vi "tdms file.vi"   [LabVIEW 2020]
uses:
  Nominal Client/Nominal Client.lvclass/Nominal Client.ctl
  nominal types/workspace/workspace.lvclass/workspace.ctl
  7420467e-f5dd-4a0f-ae77-be3a0843df19.vi
  Nominal Client/private_data.set.vi
  7420467e-f5dd-4a0f-ae77-be3a0843df19.vi/8284acbc-2d4d-4b18-b492-8ff51a6e7e10.vi
  nominal types/workspace/id.get.vi
  nominal types/workspace/rid.get.vi
  <vilib>/AdvancedString/1D String Array to Delimited String.vi
  Nominal Client/workspace.set.vi
  <vilib>/Utility/error.llb/Error Cluster From Error Code.vi
  Nominal Client/format endpoint termination.vi
  submodules/reqwest-labview/lv-src/reqwest/create.vi
  Nominal Client/workspace_cache.get_from_rid.vi
  Nominal Client/workspace_cache.get.vi
  Nominal Client/Palette Items/who_am_i.vi
  User/User.lvclass
  Nominal Client/Nominal Client.lvclass
  nominal types/workspace/workspace.lvclass
  submodules/reqwest-labview/lv-src/reqwest/reqwest.lvclass
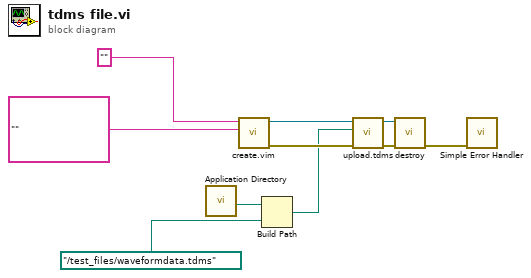
[diagram p0: block diagram]
diagram:
  n1 = call <vilib>:"Application Directory.vi"() -> ("Application Directory"=w6:path)
  n2 = call "create.vim"("Workspace"="", "API Token (string or path)"="") -> ("error out"=w7:errorcluster, "Nominal Client"=w10:refnum<class "Nominal Client.lvclass">)  [unwired: 7 in, 1 out]
  n3 = Build Path(base path=w6, name or relative path=path "../test_files/waveformdata.tdms") -> (appended path=w4:path)
  n4 = call "upload.tdms.vi"("error in"=w7, "File Path"=w4, "Nominal Client in"=w10) -> ("error out"=w8:errorcluster, "Nominal Client out"=w9:refnum<class "Nominal Client.lvclass">)  [unwired: 7 in]
  n5 = call "destroy.vi"("error in"=w8, "Nominal Client"=w9) -> ("error out"=w2:errorcluster)  [unwired: 9 in]
  n6 = call <vilib>:"Simple Error Handler.vi"("error in (no error)"=w2) -> ()  [unwired: 4 in, 5 out]
